vi "Array of U16_Static Write.vi"(8 "error in (no error)":errorcluster, 9 "Value":u16[](array[numeric]), 11 "Tag Name":string) -> (0 "error out":errorcluster)   [LabVIEW 2020, in "Current Value Table(Rebuild).lvlib"]
doc: "This VI will write the data associated with a single tag. This VI will only look up the tag index on the first call, or if the look-up resulted in an error. This VI has higher performance than the normal write function thanks to the removal of the name check."
uses:
  Current Value Table(Rebuild).lvlib
  FGVs/Tag Memory Methods.ctl
  Type Defs/Memory Commands.ctl
  Array of U16_Type To Enum.vi
  Array of U16_Memory Block.vi
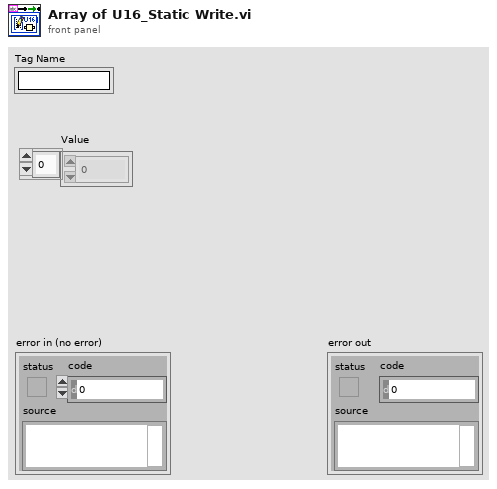
[diagram p1: front panel]
types:
  T1 = typedef "Current Value Table(Rebuild).lvlib/Tag Memory Methods.ctl" = enum16{"Clear", "Read Tag Index", "Read Tag Indices", "Generate Group", "Add Tag", "Overwrite Tag", "Read Description", "Get Stored Tags", "Write Description"}
  T2 = typedef "Current Value Table(Rebuild).lvlib/Data Types.ctl" = enum16{"Double", "Single", "I64", "I32", "I16", "I8", "U64", "U32", "U16", "U8", "String", "Boolean", "Array of U8", "Array of U16", "Array of U32", "Array of U64", "Array of I64", "Array of I32", "Array of I16", "Array of I8", "Array of Double", "Array of Single", "Array of Boolean", "Array of String"}
  T3 = typedef "Current Value Table(Rebuild).lvlib/Memory Commands.ctl" = enum16{"Init", "Add Data", "Read", "Read Group", "Read All", "Write", "Write Group", "Get Size"}
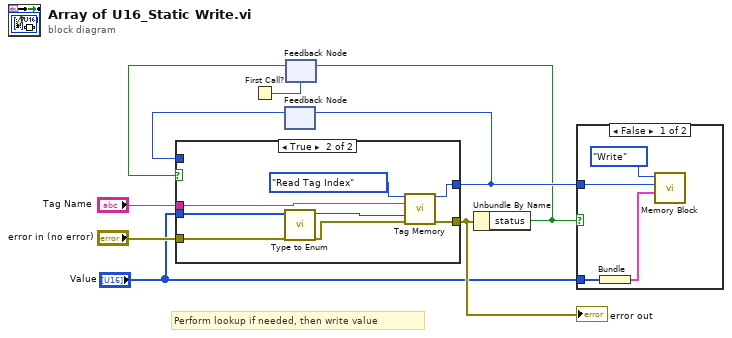
[diagram p0: block diagram]
diagram:
  # "Perform lookup if needed, then write value"
  n1 = First Call?() -> (First Call?: T/F=w2:bool)
  n2 = feedback #1() -> (w7:i32)  [unwired: 1 in]
  n3 = feedback #2(w2) -> (w3:bool)
  n4 = case shown="True" w3 {
    tunnel: [w11 w16] -> w4
    tunnel: "error in (no error)" -> [w11 w13]
    tunnel: [w10 w15] -> w9
    tunnel: w7 -> [w10 _]
    tunnel: "Tag Name" -> [_ w14]
    tunnel: "Value" -> [_ w12]
    frame False {
    }
    frame True {
      n5 = call-poly "Type to Enum.vi"("Default"=w12) -> ("Data Type Enum"=w17:T2)  [unwired: 10 in]
      n6 = call "Tag Memory.vi"("Method"=Tag_Memory_Methods."Read Tag Index", "Tag"=w14, "Expected Type"=w17, "error in (no error)"=w13) -> ("Index Out"=w15:i32, "error out"=w16:errorcluster)  [unwired: 6 in, 4 out]
    }
  }
  "error out" <- w4
  n7 = feedback-in #1(w9) -> ()
  n8 = Unbundle By Name(w4) -> ("status"=w5:bool)
  n9 = feedback-in #2(w5) -> ()
  n10 = case shown="False" w5 {
    tunnel: w9 -> [w21 _]
    tunnel: "Value" -> [w20 _]
    frame False {
      n11 = Bundle("Value"=w20) -> (w19:cluster{"Value":u16[]})  [unwired: 1 in]
      n12 = call-poly "Memory Block.vi"("Value"=w19, "Index"=w21, "Method"=Memory_Commands."Write") -> ()  [unwired: 6 in, 3 out]
    }
    frame True {
    }
  }
